vi "gwyscan generate xyz data.vi"(0 "xypos":dbl[](array[numeric]), 1 "yreal":dbl, 2 "yoffset":dbl, 5 "zdata":dbl[](array[numeric]), 7 "n":i32, 9 "xreal":dbl, 11 "error in (no error)":errorcluster, 12 "xoffset":dbl) -> (4 "xypos Out":dbl[](array[numeric]), 6 "zdata OUT":dbl[](array[numeric]), 8 "function return":i32, 15 "error out":errorcluster)   [LabVIEW 2016, in "libgwyscan.lvlib"]
doc: "GWYSCANDLL_API int gwyscan_generate_xyz_data(double *xypos, double *zdata, int n, double xreal, double yreal, double xoffset, double yoffset);\nGWYSCANDLL_API GwyscanResult gwyscan_generate_xyz_data(double *xypos, double *zdata, int n, double xreal, double yreal, double xoffset, double yoffset);"
uses:
  libgwyscan.lvlib
  libgwyscan.dll
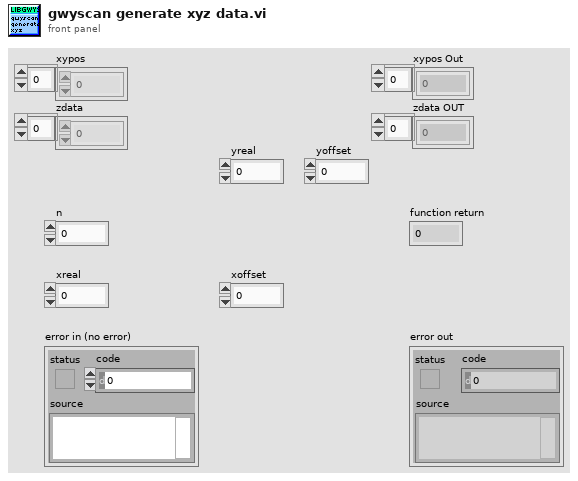
[diagram p1: front panel]
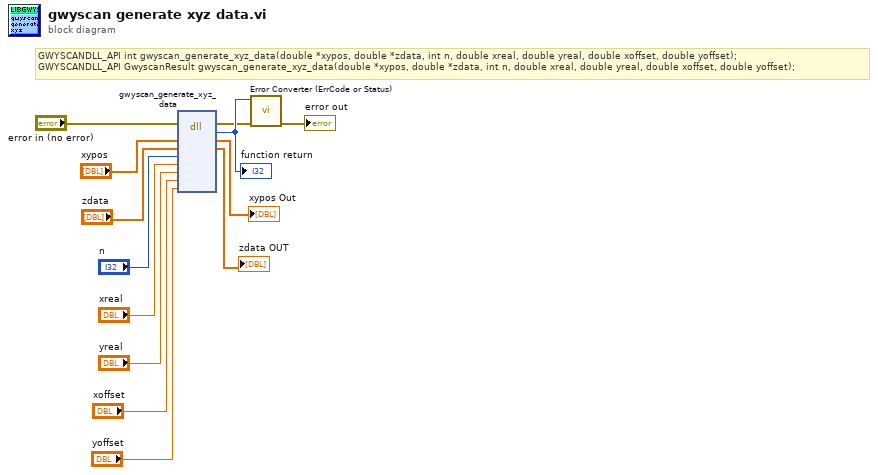
[diagram p0: block diagram]
diagram:
  # "GWYSCANDLL_API int gwyscan_generate_xyz_data(double *xypos, double *zdata, int n, double xreal, double yreal, double xoffset, double yoffset);\nGWYSCANDLL_API GwyscanResult gwyscan_generate_xyz_data(double *xypos, double *zdata, int n, double xreal, double yreal, double xoffset, double yoffset);"
  n1 = dll-call lib="PTH2abs CUsersCharlÃ¨ne BrillardDesktoplbni-lbniAFMController-BetaVersionv2.0.16-20190611 libgwyscan-1.2-labview2015-win32libgwyscan.*" fn="gwyscan_generate_xyz_data"(error in="error in (no error)", "xypos"="xypos", "zdata"="zdata", "n"="n", "xreal"="xreal", "yreal"="yreal", "xoffset"="xoffset", "yoffset"="yoffset") -> (error out=w4:errorcluster, "return type"=w13:i32, "xypos"=→"xypos Out":dbl[], "zdata"=→"zdata OUT":dbl[])  [unwired: 7 in, 1 out]
  "function return" <- w13
  n2 = call "Error Converter (ErrCode or Status).vi"("error in (no error)"=w4, "error code"=w13) -> ("error out"=→"error out":errorcluster)  [unwired: 9 in]
